vi "niRFSysCalReader Interpolator.vi"(4 "Power (dBm)":dbl, 6 "Frequency (Hz)":dbl, 8 "error in":errorcluster, 11 "niRFSysCalReader Handle":T1) -> (0 "error out":errorcluster, 2 "Interpolated Pathloss (dB)":dbl[](array[numeric]), 3 "niRFSysCalReader Handle out":T1)   [LabVIEW 2016, in "niRFSysCalReader.lvlib"]
doc: "Performs an interpolation on the Calibration Data."
uses:
  niRFSysCalReader.lvlib
  INCLUDES/niRFSysCalReader Handle.ctl
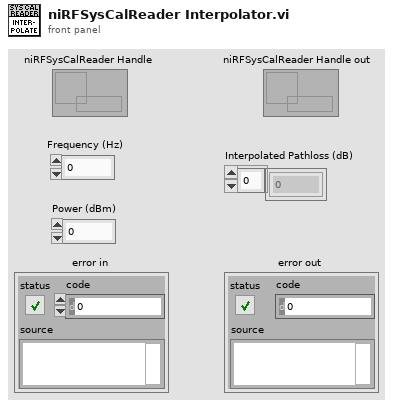
[diagram p1: front panel]
types:
  T1 = typedef "niRFSysCalReader.lvlib/niRFSysCalReader Handle.ctl" = refnum<data-value>
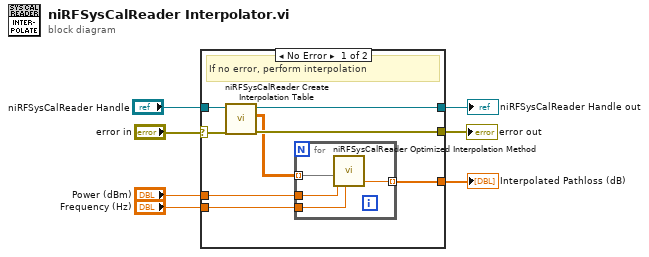
[diagram p0: block diagram]
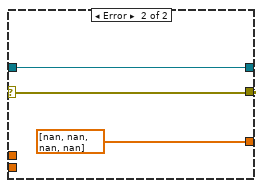
[diagram p2: hidden frame]
diagram:
  n1 = case shown="No Error" "error in" {
    selector: "error in" -> [w15 w21]
    tunnel: "Frequency (Hz)" -> [w12 _]
    tunnel: "Power (dBm)" -> [w13 _]
    tunnel: [w14 dbl[] [nan, nan, nan, nan]] -> w1
    tunnel: [w9 w21] -> w5
    tunnel: "niRFSysCalReader Handle" -> [w11 w22]
    tunnel: [w10 w22] -> w3
    frame No Error {
      # "If no error, perform interpolation"
      n2 = call "niRFSysCalReader Create Interpolation Table.vi"("error in"=w15, "niRFSysCalReader Handle"=w11) -> ("error out"=w9:errorcluster, "Interpolation Table"=w8:dbl[][][], "niRFSysCalReader Handle out"=w10:T1)  [unwired: 7 in]
      n3 = for {
        tunnel: [w19] -> w14 mode=indexing
        tunnel: w13 -> [w18]
        tunnel: w12 -> [w17]
        tunnel: w8 -> [w16] mode=indexing
        n4 = call "niRFSysCalReader Optimized Interpolation Method.vi"("Table (frequency, power, pathloss)"=w16, "Max Input Power, dBm"=w18, "Center Frequency, Hz"=w17) -> ("External Attenuation, dB"=w19:dbl)  [unwired: 2 in, 2 out]
      }
    }
    frame Error {
    }
  }
  "error out" <- w5
  "niRFSysCalReader Handle out" <- w3
  "Interpolated Pathloss (dB)" <- w1
